vi "Destroy.vi"(8 "error in (no error)":errorcluster, 10 "wait for activity?":bool, 11 "reference Class in":refnum<class "Reference Class.lvclass">) -> (0 "error out":errorcluster, 2 "final simple Class":refnum<class "Simple Class.lvclass">)   [LabVIEW 2023, in "Reference Class.lvclass"]
doc: "Use this VI to properly shut down the reference queue after you are finished with the reference object. You can also use it to perform any cleanup needed."
uses:
  Reference Class.lvclass
  SimpleClass/Simple Class.lvclass
  Reference Class.lvclass/Reference Class.ctl
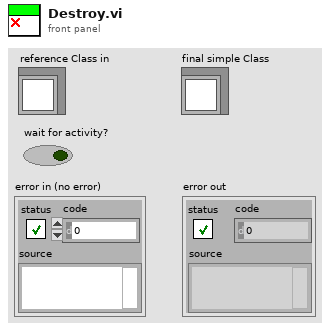
[diagram p1: front panel]
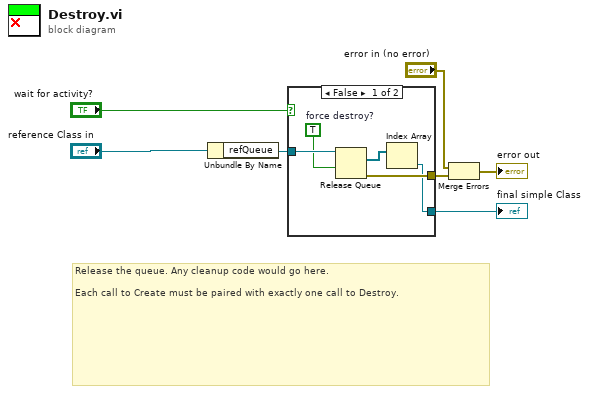
[diagram p0: block diagram]
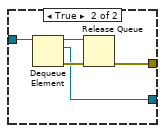
[diagram p2: hidden frame]
diagram:
  # "Release the queue. Any cleanup code would go here.\n\nEach call to Create must be paired with exactly one call to Destroy."
  n1 = Unbundle By Name("reference Class in") -> ("refQueue"=w4:refnum<queue>)
  n2 = case shown="False" "wait for activity?" {
    tunnel: w4 -> [w10 w17]
    tunnel: [w12 w14] -> w3
    tunnel: [w9 w13] -> w6
    frame False {
      w8 = TRUE  # force destroy?
      n3 = Release Queue(queue=w10, force destroy? (F)=w8) -> (remaining elements=w11:refnum<class "Simple Class.lvclass">[], error out=w12:errorcluster)  [unwired: 1 in, 1 out]
      n4 = Index Array(array=w11) -> (element=w9:refnum<class "Simple Class.lvclass">)  [unwired: 1 in]
    }
    frame True {
      n5 = Dequeue Element(queue=w17) -> (queue out=w15:refnum<queue>, element=w13:refnum<class "Simple Class.lvclass">, error out=w16:errorcluster)  [unwired: 2 in, 1 out]
      n6 = Release Queue(queue=w15, error in (no error)=w16) -> (error out=w14:errorcluster)  [unwired: 1 in, 2 out]
    }
  }
  "final simple Class" <- w6
  n7 = Merge Errors("error in (no error)", w3) -> (→"error out":errorcluster)
